vi "list_peak.vi"(11 "Position Energy":dbl format="%#_13g") -> ()   [LabVIEW 2023]
panel:
  in  "Stop Button":bool
  out "Best Match":string[][](table)
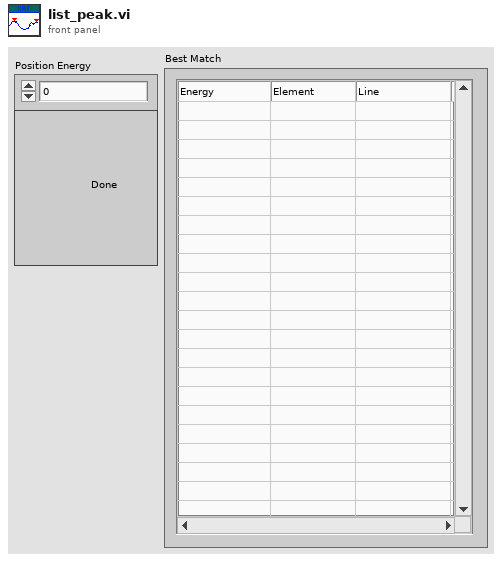
[diagram p1: front panel]
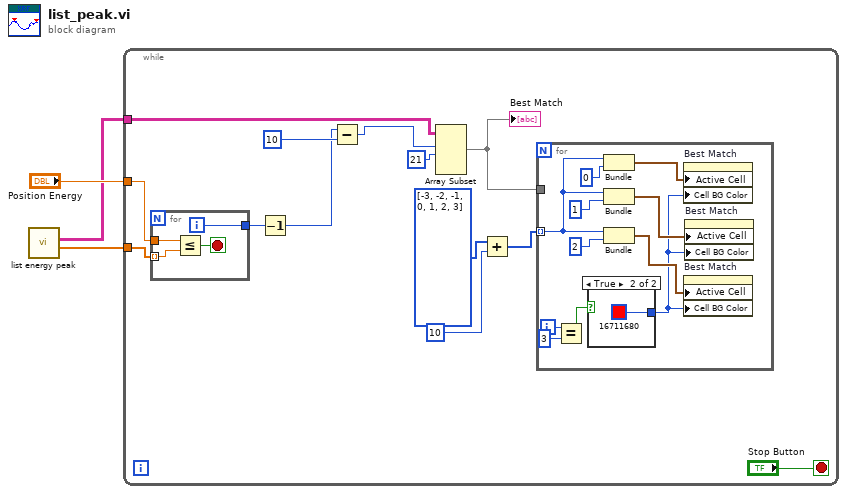
[diagram p0: block diagram]
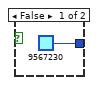
[diagram p2: hidden frame]
diagram:
  n1 = call "list energy peak.vi"() -> ("Energies Ordered"=w3:dbl[], "List Ordered"=w1:string[][])  [unwired: 6 in, 4 out]
  n2 = while {
    tunnel: w3 -> [w13]
    tunnel: "Position Energy" -> [w12]
    tunnel: w1 -> [w9]
    stop <- "Stop Button" stop-if-true
    n3 = for {
      tunnel: w12 -> [w33]
      tunnel: w13 -> [w32] mode=indexing
      tunnel: [w30] -> w16
      i -> [w30]
      stop <- w31 stop-if-true
      n4 = Less Or Equal?(x=w33, y=w32) -> (x <= y?=w31:bool)
    }
    n5 = Decrement(x=w16) -> (x-1=w14:i32)
    n6 = Subtract(x=w14, y=10) -> (x-y=w10:i32)
    n7 = Array Subset(array=w9, index (row)=w10, length (row)=21 ("length")) -> (w5:string[][])  [unwired: 2 in]
    "Best Match" <- w5
    n8 = Add(x=i32[] [-3, -2, -1, 0, 1, 2, 3], y=10) -> (x+y=w6:i32[])
    n9 = for {
      tunnel: w6 -> [w19] mode=indexing
      tunnel: w5 -> [_]
      i -> [w27]
      n10 = Equal?(x=w27, y=3) -> (x = y?=w25:bool)
      n11 = case shown="True" w25 {
        tunnel: [u32 9567230 u32 16711680] -> w17
        frame False {
        }
        frame True {
        }
      }
      n12 = Bundle(w19, 0) -> (w18:cluster{i32, i32})  [unwired: 1 in]
      n13 = Bundle(w19, 1) -> (w22:cluster{i32, i32})  [unwired: 1 in]
      n14 = Bundle(w19, 2) -> (w21:cluster{i32, i32})  [unwired: 1 in]
      n15 = property on="Best Match" class="Tbl (strict)"("Active Cell"=w18, "Cell BG Color"=w17) -> ()  [unwired: 2 in, 2 out]
      n16 = property on="Best Match" class="Tbl (strict)"("Active Cell"=w21, "Cell BG Color"=w17) -> ()  [unwired: 2 in, 2 out]
      n17 = property on="Best Match" class="Tbl (strict)"("Active Cell"=w22, "Cell BG Color"=w17) -> ()  [unwired: 2 in, 2 out]
    }
  }
